vi "Connect.vi"(7 "error in (no error)":errorcluster caption="Fehler (Eingang, kein Fehler)", 8 "ShProt?":bool, 9 "pcAComName":string, 10 "lABaudRate":i32) -> (0 "error out":errorcluster caption="Fehler (Ausgang)", 2 "function return":i32, 3 "plLSID out":i32)   [LabVIEW 2018]
uses:
  <userlib>/TANGO_DLL/Tango_DLL.lvlib
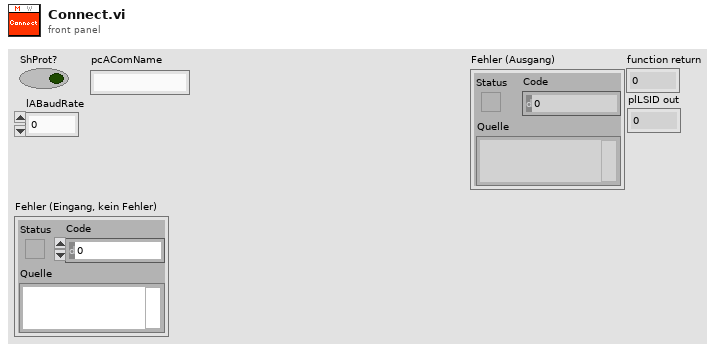
[diagram p1: front panel]
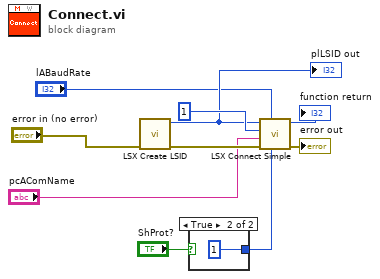
[diagram p0: block diagram]
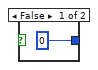
[diagram p2: hidden frame]
diagram:
  n1 = call <userlib>:"LSX Create LSID.vi"("error in (no error)"="error in (no error)") -> ("error out"=w9:errorcluster, "plLSID out"=w7:i32)  [unwired: 8 in, 1 out]
  "plLSID out" <- w7
  n2 = case shown="True" "ShProt?" {
    tunnel: [0 1] -> w8
    frame False {
    }
    frame True {
    }
  }
  n3 = call <userlib>:"LSX Connect Simple.vi"("bAShowProt"=w8, "lABaudRate"="lABaudRate", "error in (no error)"=w9, "pcAComName"="pcAComName", "lAnInterfaceType"=1, "lLSID"=w7) -> ("error out"=→"error out":errorcluster, "function return"=→"function return":i32)  [unwired: 3 in, 1 out]
